vi "_030.vi"() -> ()   [LabVIEW 2024]
panel:
  out "Boolean 7":bool
  out "Boolean 6":bool
  out "Boolean 5":bool
  out "Boolean 4":bool
  out "Boolean 3":bool
  out "Boolean 2":bool
  out "Boolean":bool
  # "7 Segment :"
  # "( Using Stacked Sequence Structure )"
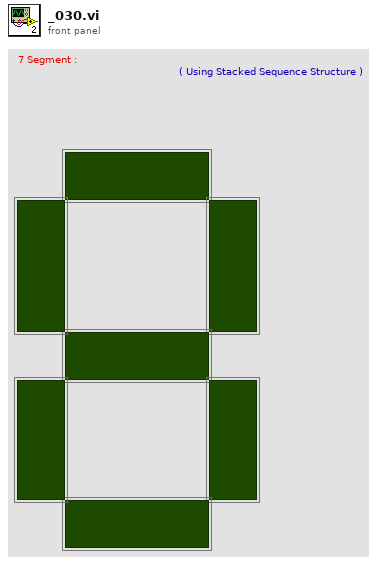
[diagram p1: front panel]
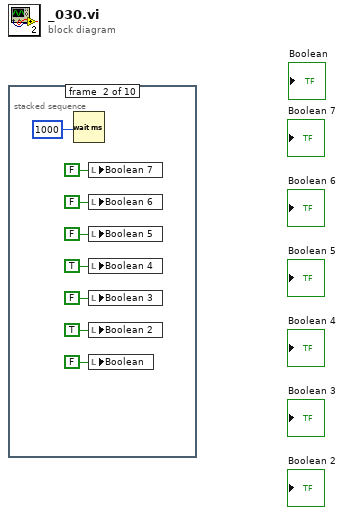
[diagram p0: block diagram]
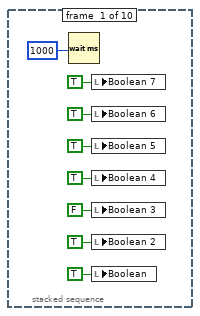
[diagram p2: hidden frame]
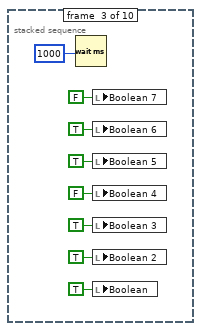
[diagram p3: hidden frame]
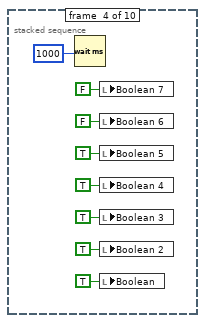
[diagram p4: hidden frame]
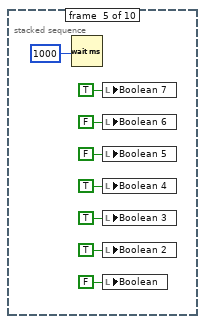
[diagram p5: hidden frame]
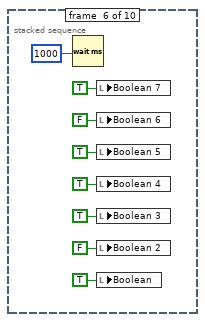
[diagram p6: hidden frame]
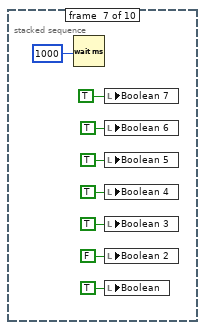
[diagram p7: hidden frame]
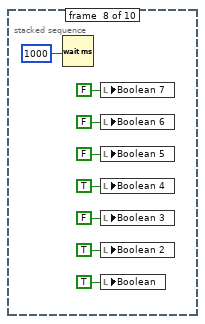
[diagram p8: hidden frame]
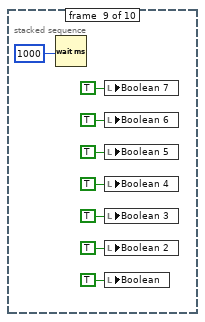
[diagram p9: hidden frame]
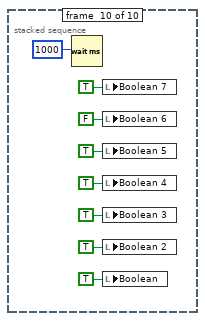
[diagram p10: hidden frame]
diagram:
  n1 = stacked-sequence {
    frame #0 {
      n2 = Wait (ms)(milliseconds to wait=u32 1000 ("millisecond timer value")) -> ()  [unwired: 1 out]
      n3 = local write "Boolean 7"(TRUE ("Boolean 7")) -> ()
      n4 = local write "Boolean 6"(TRUE ("Boolean 6")) -> ()
      n5 = local write "Boolean 5"(TRUE ("Boolean 5")) -> ()
      n6 = local write "Boolean 4"(TRUE ("Boolean 4")) -> ()
      n7 = local write "Boolean 3"(FALSE ("Boolean 3")) -> ()
      n8 = local write "Boolean 2"(TRUE ("Boolean 2")) -> ()
      n9 = local write "Boolean"(TRUE ("Boolean")) -> ()
    }
    frame #1 {
      n10 = Wait (ms)(milliseconds to wait=u32 1000 ("millisecond timer value")) -> ()  [unwired: 1 out]
      n11 = local write "Boolean 7"(FALSE ("Boolean 7")) -> ()
      n12 = local write "Boolean 6"(FALSE ("Boolean 6")) -> ()
      n13 = local write "Boolean 5"(FALSE ("Boolean 5")) -> ()
      n14 = local write "Boolean 4"(TRUE ("Boolean 4")) -> ()
      n15 = local write "Boolean 3"(FALSE ("Boolean 3")) -> ()
      n16 = local write "Boolean 2"(TRUE ("Boolean 2")) -> ()
      n17 = local write "Boolean"(FALSE ("Boolean")) -> ()
    }
    frame #2 {
      n18 = Wait (ms)(milliseconds to wait=u32 1000 ("millisecond timer value")) -> ()  [unwired: 1 out]
      n19 = local write "Boolean 7"(FALSE ("Boolean 7")) -> ()
      n20 = local write "Boolean 6"(TRUE ("Boolean 6")) -> ()
      n21 = local write "Boolean 5"(TRUE ("Boolean 5")) -> ()
      n22 = local write "Boolean 4"(FALSE ("Boolean 4")) -> ()
      n23 = local write "Boolean 3"(TRUE ("Boolean 3")) -> ()
      n24 = local write "Boolean 2"(TRUE ("Boolean 2")) -> ()
      n25 = local write "Boolean"(TRUE ("Boolean")) -> ()
    }
    frame #3 {
      n26 = Wait (ms)(milliseconds to wait=u32 1000 ("millisecond timer value")) -> ()  [unwired: 1 out]
      n27 = local write "Boolean 7"(FALSE ("Boolean 7")) -> ()
      n28 = local write "Boolean 6"(FALSE ("Boolean 6")) -> ()
      n29 = local write "Boolean 5"(TRUE ("Boolean 5")) -> ()
      n30 = local write "Boolean 4"(TRUE ("Boolean 4")) -> ()
      n31 = local write "Boolean 3"(TRUE ("Boolean 3")) -> ()
      n32 = local write "Boolean 2"(TRUE ("Boolean 2")) -> ()
      n33 = local write "Boolean"(TRUE ("Boolean")) -> ()
    }
    frame #4 {
      n34 = Wait (ms)(milliseconds to wait=u32 1000 ("millisecond timer value")) -> ()  [unwired: 1 out]
      n35 = local write "Boolean 7"(TRUE ("Boolean 7")) -> ()
      n36 = local write "Boolean 6"(FALSE ("Boolean 6")) -> ()
      n37 = local write "Boolean 5"(FALSE ("Boolean 5")) -> ()
      n38 = local write "Boolean 4"(TRUE ("Boolean 4")) -> ()
      n39 = local write "Boolean 3"(TRUE ("Boolean 3")) -> ()
      n40 = local write "Boolean 2"(TRUE ("Boolean 2")) -> ()
      n41 = local write "Boolean"(FALSE ("Boolean")) -> ()
    }
    frame #5 {
      n42 = Wait (ms)(milliseconds to wait=u32 1000 ("millisecond timer value")) -> ()  [unwired: 1 out]
      n43 = local write "Boolean 7"(TRUE ("Boolean 7")) -> ()
      n44 = local write "Boolean 6"(FALSE ("Boolean 6")) -> ()
      n45 = local write "Boolean 5"(TRUE ("Boolean 5")) -> ()
      n46 = local write "Boolean 4"(TRUE ("Boolean 4")) -> ()
      n47 = local write "Boolean 3"(TRUE ("Boolean 3")) -> ()
      n48 = local write "Boolean 2"(FALSE ("Boolean 2")) -> ()
      n49 = local write "Boolean"(TRUE ("Boolean")) -> ()
    }
    frame #6 {
      n50 = Wait (ms)(milliseconds to wait=u32 1000 ("millisecond timer value")) -> ()  [unwired: 1 out]
      n51 = local write "Boolean 7"(TRUE ("Boolean 7")) -> ()
      n52 = local write "Boolean 6"(TRUE ("Boolean 6")) -> ()
      n53 = local write "Boolean 5"(TRUE ("Boolean 5")) -> ()
      n54 = local write "Boolean 4"(TRUE ("Boolean 4")) -> ()
      n55 = local write "Boolean 3"(TRUE ("Boolean 3")) -> ()
      n56 = local write "Boolean 2"(FALSE ("Boolean 2")) -> ()
      n57 = local write "Boolean"(TRUE ("Boolean")) -> ()
    }
    frame #7 {
      n58 = Wait (ms)(milliseconds to wait=u32 1000 ("millisecond timer value")) -> ()  [unwired: 1 out]
      n59 = local write "Boolean 7"(FALSE ("Boolean 7")) -> ()
      n60 = local write "Boolean 6"(FALSE ("Boolean 6")) -> ()
      n61 = local write "Boolean 5"(FALSE ("Boolean 5")) -> ()
      n62 = local write "Boolean 4"(TRUE ("Boolean 4")) -> ()
      n63 = local write "Boolean 3"(FALSE ("Boolean 3")) -> ()
      n64 = local write "Boolean 2"(TRUE ("Boolean 2")) -> ()
      n65 = local write "Boolean"(TRUE ("Boolean")) -> ()
    }
    frame #8 {
      n66 = Wait (ms)(milliseconds to wait=u32 1000 ("millisecond timer value")) -> ()  [unwired: 1 out]
      n67 = local write "Boolean 7"(TRUE ("Boolean 7")) -> ()
      n68 = local write "Boolean 6"(TRUE ("Boolean 6")) -> ()
      n69 = local write "Boolean 5"(TRUE ("Boolean 5")) -> ()
      n70 = local write "Boolean 4"(TRUE ("Boolean 4")) -> ()
      n71 = local write "Boolean 3"(TRUE ("Boolean 3")) -> ()
      n72 = local write "Boolean 2"(TRUE ("Boolean 2")) -> ()
      n73 = local write "Boolean"(TRUE ("Boolean")) -> ()
    }
    frame #9 {
      n74 = Wait (ms)(milliseconds to wait=u32 1000 ("millisecond timer value")) -> ()  [unwired: 1 out]
      n75 = local write "Boolean 7"(TRUE ("Boolean 7")) -> ()
      n76 = local write "Boolean 6"(FALSE ("Boolean 6")) -> ()
      n77 = local write "Boolean 5"(TRUE ("Boolean 5")) -> ()
      n78 = local write "Boolean 4"(TRUE ("Boolean 4")) -> ()
      n79 = local write "Boolean 3"(TRUE ("Boolean 3")) -> ()
      n80 = local write "Boolean 2"(TRUE ("Boolean 2")) -> ()
      n81 = local write "Boolean"(TRUE ("Boolean")) -> ()
    }
  }
